vi "XY Graph Compute Sliced Mean, SDV & CV Plots.vi"(8 "error in (no error)":errorcluster, 10 "Plot":cluster{"X Array":dbl[], "Y Array":dbl[]}, 11 "Slices Definition":T1={"Axis Start"=0.0, "Axis Stop"=0.0, "# Steps"=0, "Step Size"=1.0, "Step Definition"=enum."# Steps", "Upper Percentile"=1.0, "Lower Percentile"=1.0, "Min # Data Points/Slice"=1, "Output Abscissa Statistics Plots"=FALSE, "Bin Location"=enum."Left"} {"Min # Data Points/Slice" min=0 max=100; "Lower Percentile" min=0.0 max=100.0; "Upper Percentile" min=0.0 max=100.0; "Step Size" min=1.0; "# Steps" min=1}) -> (0 "error out":errorcluster, 2 "Bin Intensity Distribution":cluster{"Intensity Array":sgl[]}[](array[cluster]), 3 "Plots":cluster{"X Array":dbl[], "Y Array":dbl[]}[](array[cluster]))   [LabVIEW 2021, in "XY Graph Add-Ons.lvlib"]
uses:
  XY Graph Add-Ons.lvlib
  XY Graph Sliced Mean & SDV Step Definition.ctl
  XY Graph Sliced CV Abscissa Location.ctl
  Arrays/Linear Ramp End Options.ctl
  49f03c9f-9bb8-4480-9460-08b8970c46f1.vi
  f2368cde-c411-4778-92ad-cdfa6392accb.vi
  ad4c9e8f-85ce-46f2-8889-cace00dc3fba.vi
  <userlib>/_OpenG.lib/array/array.llb/Sort 1D Array (DBL)__ogtk.vi
  <vilib>/Utility/error.llb/Error Cluster From Error Code.vi
  <vilib>/ErrorRing/Error Ring.xnode
  <userlib>/_OpenG.lib/array/array.llb/Reorder 1D Array2 (DBL)__ogtk.vi
  <vilib>/gmath/statdist.llb/st_Percentiles (array).vi
  Arrays/Arrays.lvlib
  <userlib>/_OpenG.lib/array/array.llb/openg_array.lvlib
  <vilib>/gmath/NI_Gmath.lvlib
  Comparison/Comparison.lvlib
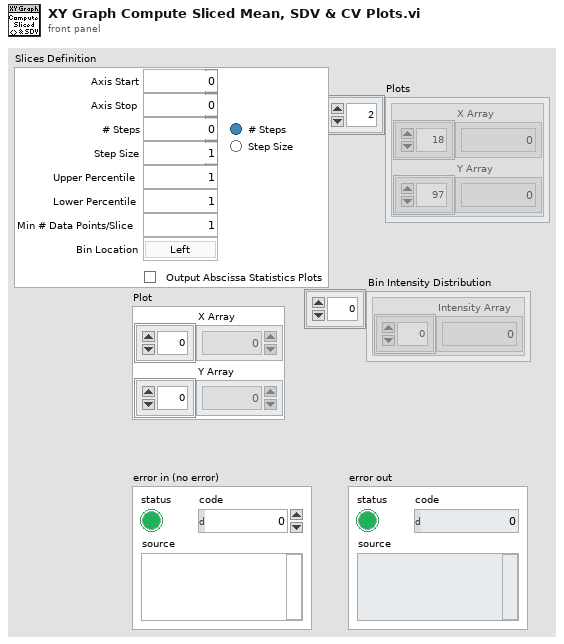
[diagram p1: front panel]
types:
  T1 = typedef "XY Graph Add-Ons.lvlib/XY Graph Sliced Mean & SDV Step Definition.ctl" = cluster{"Axis Start":dbl, "Axis Stop":dbl, "# Steps":i32, "Step Size":dbl, "Step Definition":enum32{"# Steps", "Step Size"}, "Upper Percentile":dbl, "Lower Percentile":dbl, "Min # Data Points/Slice":i32, "Output Abscissa Statistics Plots":bool, "Bin Location":T2}
  T2 = typedef "XY Graph Add-Ons.lvlib/XY Graph Sliced CV Abscissa Location.ctl" = enum16{"Left", "Center", "Mean", "Right"}
  T3 = typedef "Arrays.lvlib/Linear Ramp End Options.ctl" = enum16{"Include Min/Exclude Max", "Exclude Min/Include Max", "Include Both Ends", "Exclude Both Ends"}
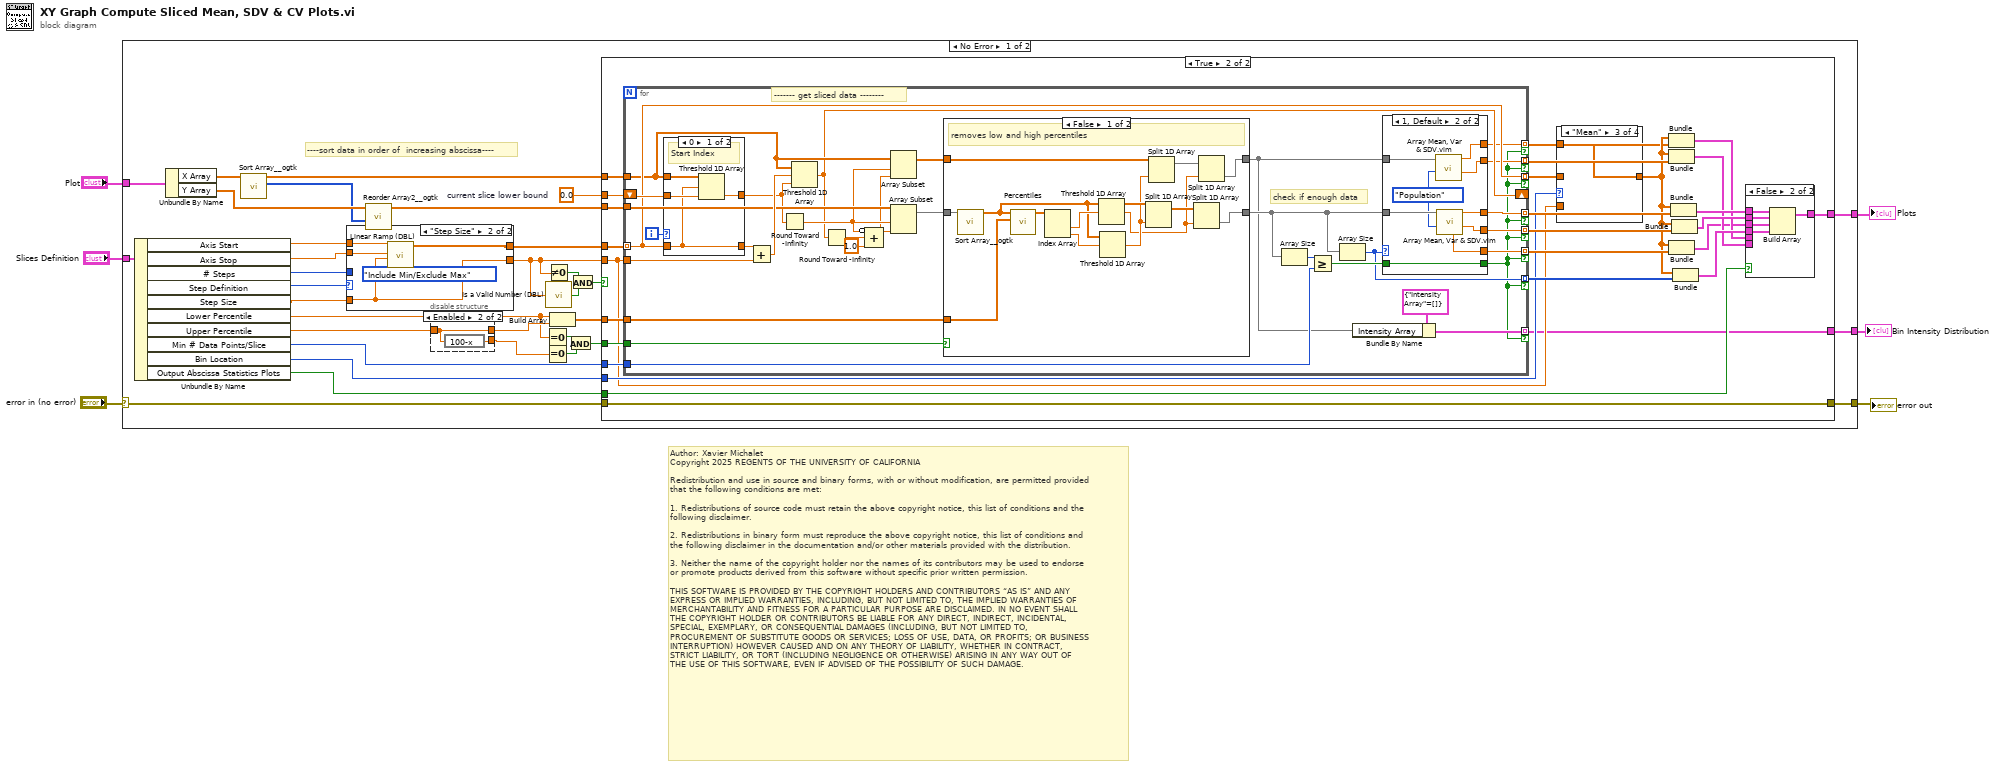
[diagram p0: block diagram]
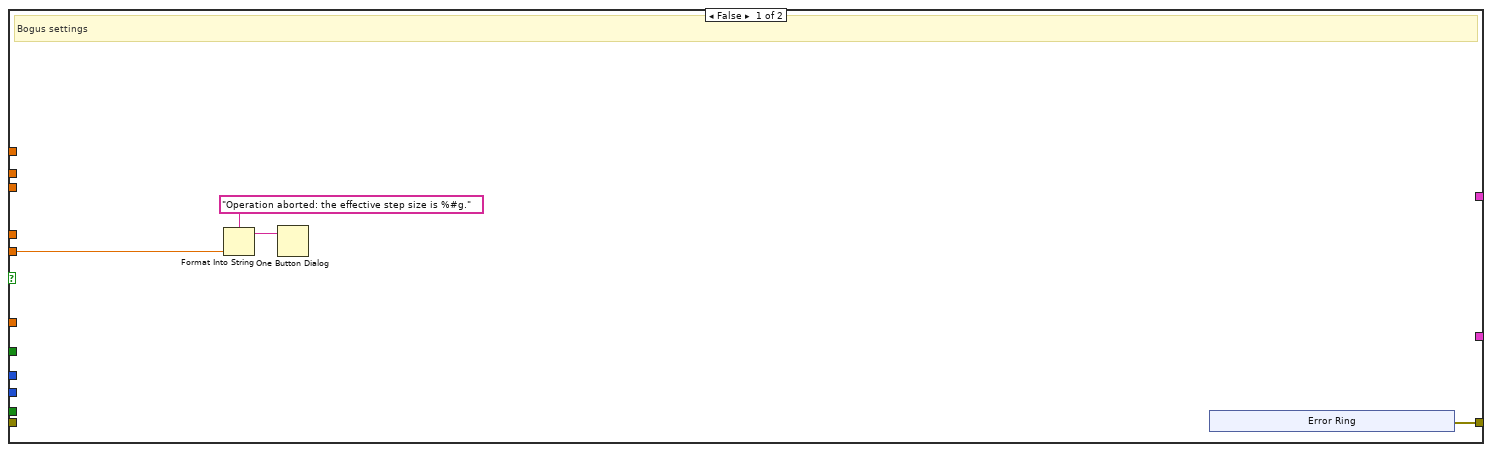
[diagram p2: hidden frame]
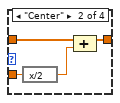
[diagram p4: hidden frame]
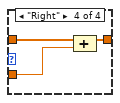
[diagram p5: hidden frame]
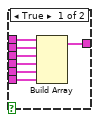
[diagram p6: hidden frame]
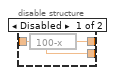
[diagram p10: hidden frame]
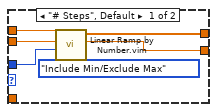
[diagram p11: hidden frame]
diagram:
  # "Author: Xavier Michalet\nCopyright 2025 REGENTS OF THE UNIVERSITY OF CALIFORNIA\n\nRedistribution and use in source and binary forms, with or without modification, are permitted provided\nthat the following conditions are met:\n\n1. Redistributions of source code must retain the above copyright notice, this list of conditions and the\nfollowing disclaimer.\n\n2. Redistributions in binary form must reproduce the above copyright notice, this list of conditions and\nthe following disclaimer in the documentation and/or other materials provided with the distribution.\n\n3. Neither the name of the copyright holder nor the names of its contributors may be used to endorse \nor promote products derived from this software without specific prior written permission.\n\nTHIS SOFTWARE IS PROVIDED BY THE COPYRIGHT HOLDERS AND CONTRIBUTORS “AS IS” AND ANY \nEXPRESS OR IMPLIED WARRANTIES, INCLUDING, BUT NOT LIMITED TO, THE IMPLIED WARRANTIES OF\nMERCHANTABILITY AND FITNESS FOR A PARTICULAR PURPOSE ARE DISCLAIMED. IN NO EVENT SHALL\nTHE COPYRIGHT HOLDER OR CONTRIBUTORS BE LIABLE FOR ANY DIRECT, INDIRECT, INCIDENTAL, \nSPECIAL, EXEMPLARY, OR CONSEQUENTIAL DAMAGES (INCLUDING, BUT NOT LIMITED TO, \nPROCUREMENT OF SUBSTITUTE GOODS OR SERVICES; LOSS OF USE, DATA, OR PROFITS; OR BUSINESS\nINTERRUPTION) HOWEVER CAUSED AND ON ANY THEORY OF LIABILITY, WHETHER IN CONTRACT, \nSTRICT LIABILITY, OR TORT (INCLUDING NEGLIGENCE OR OTHERWISE) ARISING IN ANY WAY OUT OF\nTHE USE OF THIS SOFTWARE, EVEN IF ADVISED OF THE POSSIBILITY OF SUCH DAMAGE."
  n1 = case shown="No Error" "error in (no error)" {
    selector: "error in (no error)" -> [w10 w173]
    tunnel: "Plot" -> [w39 _]
    tunnel: "Slices Definition" -> [w38 _]
    tunnel: [w28 _] -> w4
    tunnel: [w9 w173] -> w2
    tunnel: [w7 _] -> w1
    frame No Error {
      w29 = 0.0  # current slice lower bound
      # "----sort data in order of  increasing abscissa----"
      n2 = Unbundle By Name(w38) -> ("Axis Start"=w37:dbl, "Axis Stop"=w36:dbl, "# Steps"=w35:i32, "Step Definition"=w27:enum32{"# Steps", "Step Size"}, "Step Size"=w26:dbl, "Lower Percentile"=w22:dbl, "Upper Percentile"=w17:dbl, "Min # Data Points/Slice"=w20:i32, "Bin Location"=w8:T2, "Output Abscissa Statistics Plots"=w15:bool)
      n3 = Unbundle By Name(w39) -> ("X Array"=w34:dbl[], "Y Array"=w33:dbl[])
      n4 = call-poly <userlib>:"Sort Array__ogtk.vi"("Array in"=w34) -> ("Sorted Pointers"=w32:i32[], "Sorted Array out"=w31:dbl[])  [unwired: 9 in]
      n5 = case shown="\"Step Size\"" w27 {
        tunnel: w37 -> [w167 w172]
        tunnel: w36 -> [w166 w171]
        tunnel: w35 -> [w165 _]
        tunnel: [w163 w168] -> w14
        tunnel: [w162 w169] -> w25
        tunnel: w26 -> [_ w168]
        frame "# Steps", Default {
          n6 = call "Linear Ramp by Number.vim"("Options"=Linear_Ramp_End_Options."Include Min/Exclude Max", "# Steps (1)"=w165, "End (1)"=w166, "Start (0)"=w167) -> ("Step Size"=w163:dbl, "Ramp"=w162:dbl[])  [unwired: 5 in, 1 out]
        }
        frame "Step Size" {
          n7 = call "Linear Ramp (DBL).vi"("Options"=Linear_Ramp_End_Options."Include Min/Exclude Max", "Delta"=w168, "Max"=w171, "Min"=w172) -> ("Ramp"=w169:dbl[])  [unwired: 6 in, 1 out]
        }
      }
      n8 = call-poly <userlib>:"Reorder Array2__ogtk.vi"("indices"=w32, "array"=w33) -> ("reordered array"=w30:dbl[])  [unwired: 9 in]
      n9 = disable-structure shown="Enabled" {
        disable-tunnel: [w159 w160] -> w23
        disable-tunnel: w17 -> [w158 w160]
        disable-tunnel: [w158 w161] -> w16
        frame Disabled {
          n10 = expression code="100-x"(w158) -> (w159:dbl)
        }
        frame Enabled {
          n11 = expression code="100-x"(w160) -> (w161:dbl)
        }
      }
      n12 = Equal To 0?(x=w22) -> (x = 0?=w21:bool)
      n13 = Equal To 0?(x=w16) -> (x = 0?=w19:bool)
      n14 = call "Is a Valid Number (DBL).vi"("Number"=w14) -> ("Valid Number?"=w12:bool)  [unwired: 8 in]
      n15 = Not Equal To 0?(x=w14) -> (x != 0?=w13:bool)
      n16 = Build Array(w22, w23) -> (w24:dbl[])
      n17 = And(x=w21, y=w19) -> (x .and. y?=w18:bool)
      n18 = And(x=w13, y=w12) -> (x .and. y?=w11:bool)
      n19 = case shown="True" w11 {
        tunnel: w31 -> [_ w74]
        tunnel: w30 -> [_ w73]
        tunnel: w29 -> [_ w72]
        tunnel: [_ w67] -> w28
        tunnel: w25 -> [_ w66]
        tunnel: w24 -> [_ w63]
        tunnel: w20 -> [_ w62]
        tunnel: w18 -> [_ w61]
        tunnel: w15 -> [_ w57]
        tunnel: w14 -> [w41 w50]
        tunnel: w10 -> [_ w56]
        tunnel: [w40 w56] -> w9
        tunnel: w8 -> [_ w52]
        tunnel: [_ w48] -> w7
        frame False {
          # "Bogus settings"
          n20 = Format Into String(format string="Operation aborted: the effective step size is %#g.", w41) -> (resulting string=w43:string)  [unwired: 2 in, 1 out]
          n21 = One Button Dialog(message=w43) -> ()  [unwired: 1 in, 1 out]
          n22 = xnode "Error Ring"() -> ("error out"=w40:errorcluster)
        }
        frame True {
          n23 = for {
            tunnel: w66 -> [w113] mode=indexing
            tunnel: w74 -> [w108]
            tunnel: w73 -> [w122]
            shift-right: [w104] -> _
            shift-left: w72 -> [w126]
            tunnel: w50 -> [w124]
            tunnel: [w118] -> w71 mode=indexing if=w96
            tunnel: [w117] -> w70 mode=indexing if=w96
            tunnel: [w101] -> w65 mode=indexing if=w96
            tunnel: w63 -> [w116]
            tunnel: w62 -> [w114]
            tunnel: [w113] -> w53 mode=indexing if=w96
            tunnel: w61 -> [w109]
            tunnel: [w103] -> w49 mode=indexing if=w96
            tunnel: [w102] -> w60 mode=indexing if=w96
            tunnel: [w100] -> w55 mode=indexing if=w96
            tunnel: [w97] -> w48 mode=indexing if=w96
            i -> [w127]
            # "------- get sliced data --------"
            # "check if enough data"
            n24 = case shown="0" w127 {
              tunnel: w108 -> [w155 _]
              tunnel: w113 -> [w152 w157]
              tunnel: w126 -> [w154 w156]
              tunnel: [w153 w156] -> w121
              tunnel: [w152 w157] -> w125
              frame 0 {
                # "Start Index"
                n25 = Threshold 1D Array(1:w154, 2:w152, 3:w155) -> (0:w153:dbl)
              }
              frame 1, Default {
              }
            }
            n26 = Add(x=w125, y=w124) -> (x+y=w123:dbl)
            n27 = Round Toward -Infinity(1:w121) -> (0:w107:dbl)
            n28 = Threshold 1D Array(1:w121, 2:w123, 3:w108) -> (0:w104:dbl)
            n29 = Round Toward -Infinity(1:w104) -> (0:w120:dbl)
            n30 = Compound Arithmetic op=ADD(invert w107, w120, 1.0 ("value")) -> (w106:dbl)
            n31 = Array Subset(array=w108, index=w107, length=w106) -> (w105:dbl[])
            n32 = Array Subset(array=w122, index=w107, length=w106) -> (w110:dbl[])
            n33 = case shown="False" w109 {
              tunnel: w116 -> [w140 _]
              tunnel: [w138 w142] -> w115
              tunnel: w110 -> [w134 w142]
              tunnel: w105 -> [w132 w141]
              tunnel: [w129 w141] -> w98
              frame False {
                # "removes low and high percentiles"
                n34 = call-poly <userlib>:"Sort Array__ogtk.vi"("Array in"=w134) -> ("Sorted Array out"=w133:dbl[])  [unwired: 9 in, 1 out]
                n35 = call-poly <vilib>:"Percentiles.vi"("p array"=w140, "x array"=w133) -> ("percentiles"=w139:dbl[])  [unwired: 8 in, 1 out]
                n36 = Index Array(array=w139) -> (element #1=w137:dbl, element #2=w135:dbl)  [unwired: 2 in]
                n37 = Threshold 1D Array(2:w137, 3:w133) -> (0:w128:dbl)  [unwired: 1 in]
                n38 = Threshold 1D Array(2:w135, 3:w133) -> (0:w131:dbl)  [unwired: 1 in]
                n39 = Split 1D Array(array=w133, index=w131) -> (first subarray=w136:dbl[])  [unwired: 1 out]
                n40 = Split 1D Array(array=w132, index=w131) -> (first subarray=w130:dbl[])  [unwired: 1 out]
                n41 = Split 1D Array(array=w136, index=w128) -> (second subarray=w138:dbl[])  [unwired: 1 out]
                n42 = Split 1D Array(array=w130, index=w128) -> (second subarray=w129:dbl[])  [unwired: 1 out]
              }
              frame True {
                # "Do not reject outliers"
              }
            }
            n43 = Array Size(array=w115) -> (size(s)=w111:i32)
            n44 = Greater Or Equal?(x=w111, y=w114) -> (x >= y?=w112:bool)
            n45 = Array Size(array=w115) -> (size(s)=w101:i32)
            n46 = Bundle By Name(cluster=cluster{"Intensity Array":sgl[]} {"Intensity Array"=[]} ("Cluster"), "Intensity Array"=w98) -> (w97:cluster{"Intensity Array":sgl[]})
            n47 = case shown="1, Default" w101 {
              tunnel: [_ w151] -> w118
              tunnel: [_ w150] -> w117
              tunnel: w115 -> [_ w149]
              tunnel: w112 -> [_ w148]
              tunnel: [_ w148] -> w96
              tunnel: w98 -> [_ w147]
              tunnel: [_ w145] -> w103
              tunnel: [_ w144] -> w102
              tunnel: [_ w143] -> w100
              frame 0 {
              }
              frame 1, Default {
                w146 = enum16{"Sample", "Population"}."Population" ("Weighting (Sample)")
                n48 = call "Array Mean, Var & SDV.vim"("Weighting (Sample)"=w146, "Array"=w147) -> ("Array SDV"=w144:dbl, "Array Mean"=w145:dbl)  [unwired: 5 in, 3 out]
                n49 = call "Array Mean, Var & SDV.vim"("Weighting (Sample)"=w146, "Array"=w149) -> ("Array SDV"=w150:dbl, "Array Mean"=w151:dbl, "Array CV"=w143:dbl)  [unwired: 5 in, 2 out]
              }
            }
          }
          n50 = case shown="\"Mean\"" w52 {
            tunnel: w53 -> [w75 w79 _ w83]
            tunnel: [w75 w76 w80 w82] -> w51
            tunnel: w50 -> [_ w78 _ w81]
            tunnel: w49 -> [_ _ w80 _]
            frame "Left", Default {
            }
            frame "Center" {
              n51 = expression code="x/2"(w78) -> (w77:dbl)
              n52 = Compound Arithmetic op=ADD(w79, w77) -> (w76:dbl[])
            }
            frame "Mean" {
            }
            frame "Right" {
              n53 = Compound Arithmetic op=ADD(w83, w81) -> (w82:dbl[])
            }
          }
          n54 = Bundle(w51, w49) -> (w59:cluster{dbl[], dbl[]})  [unwired: 1 in]
          n55 = Bundle(w51, w60) -> (w58:cluster{dbl[], dbl[]})  [unwired: 1 in]
          n56 = Bundle(w51, w55) -> (w54:cluster{dbl[], dbl[]})  [unwired: 1 in]
          n57 = Bundle(w51, w71) -> (w69:cluster{dbl[], dbl[]})  [unwired: 1 in]
          n58 = Bundle(w51, w70) -> (w68:cluster{dbl[], dbl[]})  [unwired: 1 in]
          n59 = Bundle(w51, w65) -> (w64:cluster{dbl[], i32[]})  [unwired: 1 in]
          n60 = case shown="False" w57 {
            tunnel: w69 -> [w90 w95]
            tunnel: w68 -> [w89 w94]
            tunnel: [w88 w93] -> w67
            tunnel: w64 -> [w85 w92]
            tunnel: w59 -> [w87 _]
            tunnel: w58 -> [w86 _]
            tunnel: w54 -> [w84 w91]
            frame True {
              n61 = Build Array(w90, w89, w84, w85, w87, w86) -> (w88:cluster{dbl[], dbl[]}[])
            }
            frame False {
              n62 = Build Array(w95, w94, w91, w92) -> (w93:cluster{dbl[], dbl[]}[])
            }
          }
        }
      }
    }
    frame Error {
    }
  }
  "error out" <- w2
  "Plots" <- w4
  "Bin Intensity Distribution" <- w1
